vi "FPGA-HS-Parallel-Port-Receiver.vi"() -> ()   [LabVIEW 2016]
uses:
  <vilib>/Platform/TimedLoop/XDataNode/timing_clust.ctl
  <vilib>/Platform/TimedLoop/XDataNode/nitl_modes.ctl
  <vilib>/Platform/TimedLoop/XDataNode/wakeup.ctl
  <vilib>/rvi/Emulation/niFpgaGetClockAttributes.vi
  <vilib>/rvi/Emulation/niFpgaSctlEmulationGetInTimedLoop.vi
  <vilib>/rvi/Emulation/niFpgaEmulationReportErrorSimple.vi
  <vilib>/rvi/Emulation/niFpgaCriticalErrorInLSC.vi
  <vilib>/rvi/eio/common/nirviEmuTemplateMethod_errors.vi
  <vilib>/rvi/interface/RandomDataEmulation/niFpgaRandomDataHandleErrors.vi
  <vilib>/Platform/TimedLoop/XDataNode/XDataNode.xnode
  <vilib>/eio/EIONode/EIONode.xnode
  <vilib>/rvi/DataTransferAndStorage/Container/XNode/niFpgaContainer.xnode
  <vilib>/rvi/interface/RandomDataEmulation/nirviRandomDataFpgaReadWriteTemplate.vi
  <vilib>/Platform/TimedLoop/XDataNode/XDNodeRunTimeDep.lvlib
panel:
  out "CompareVal":u16
  out "OldVal":u16
  in  "StepSize":u16=1
  in  "CompArray":u16[](array[numeric])=[0, 1, 2, 3, 4, 5, 6, 7, 8, 9, 10, 11, 12, 13, 14, 15, 16, 17, 18, 19, 20, 21, 22, 23, 24, 25, 26, 27, 28, 29, 30, 31, 32, 33, 34, 35, 36, 37, 38, 39, 40, 41, 42, 43, 44, 45, 46, 47, 48, 49, 50, 51, 52, 53, 54, 55, 56, 57, 58, 59, 60, 61, 62, 63] format="%x"
  in  "StopOnError?":bool
  out "CurrentIndex":u16 format="%x"
  out "CurrentSample":u16 format="%x"
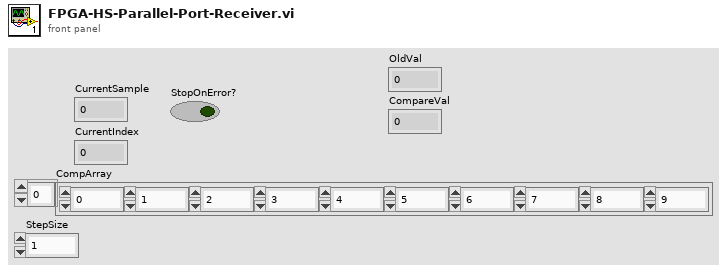
[diagram p1: front panel]
types:
  T1 = typedef "XDNodeRunTimeDep.lvlib/timing_clust.ctl" = cluster{"Expected End [f-1]":u64, "Actual End [f-1]":u64, "Finished Late? [f-1]":bool, "Expected End [i-1]":u64, "Actual End [i-1]":u64, "Finished Late? [i-1]":bool, "Expected Start [i]":u64, "Actual Start [i]":u64, "Expected Start [f]":u64, "Actual Start [f]":u64, "Source Name":string, "Structure Name":string, "Period":i64, "Deadline":i64, "Offset":i64, "Start":i64, "Priority":i32, "Timeout":i32, "Mode":T2, "Wakeup Reason":T3, "Error":errorcluster, "Source Type":string, "Secondary Source Type":string, "Global End Time":u64, "Global Start Time":u64, "Frame Duration":u64, "Iteration Duration":u64, "Assigned CPU":i32, "I/O Scan Engine Mode":u32}
  T2 = typedef "XDNodeRunTimeDep.lvlib/nitl_modes.ctl" = enum32{"No Change", "Process missed periods, maintain original phase", "Discard missed periods, maintain original phase", "Process missed periods, ignore original phase", "Discard missed periods, ignore original phase"}
  T3 = typedef "XDNodeRunTimeDep.lvlib/wakeup.ctl" = enum32{"Normal", "Aborted", "Asynchronous wakeup", "Timing source error", "Timed loop error", "Timeout"}
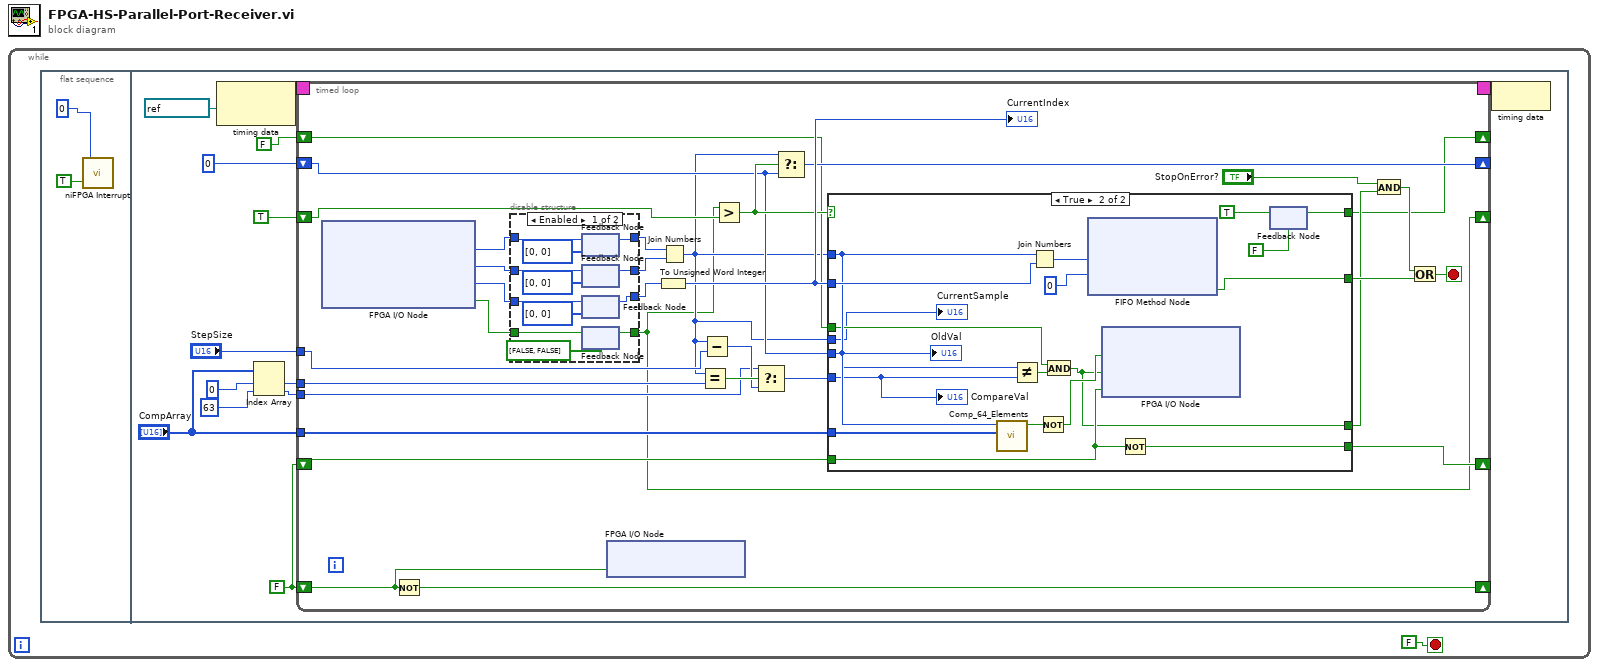
[diagram p0: block diagram]
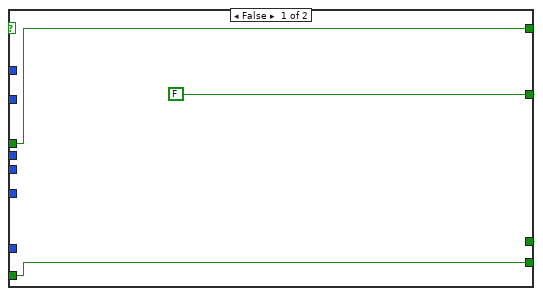
[diagram p3: hidden frame]
diagram:
  n1 = while {
    stop <- FALSE stop-if-true
    n2 = flat-sequence {
      frame #0 {
        n3 = call <vilib>:"niFPGA Interrupt.vi"("Wait Until Cleared (F)"=TRUE, "IRQ Number (0)"=u8 0) -> ()  [unwired: 1 in]
      }
      frame #1 {
        w4 = FALSE ("ConnectorB/DIO8")
        n4 = node-c288(refnum<k21> "30MHz" ("Source Name")) -> (w16:T1)
        n5 = Index Array(array="CompArray", index #1=0 ("index"), index #2=63 ("index")) -> (element #1=w8:u16, element #2=w7:u16)
        n6 = timed-loop {
          timing: w16 -> [_]
          timing-out: [_] -> w15
          shift-right: [w17] -> _
          shift-left: TRUE ("ConnectorB/DIO8") -> [w47]
          shift-right: [w46] -> _
          shift-left: w4 -> [w40]
          tunnel: "CompArray" -> [w38]
          tunnel: "StepSize" -> [w35]
          shift-right: [w32] -> _
          shift-left: u16 0 -> [w30]
          tunnel: w8 -> [w34]
          tunnel: w7 -> [w33]
          shift-right: [w28] -> _
          shift-left: FALSE -> [w29]
          shift-right: [w26] -> _
          shift-left: w4 -> [w27]
          stop <- w45 stop-if-true
          n7 = xnode "FPGA I/O Node"() -> ("ConnectorA/DIO15:8"=w24:u8, "ConnectorA/DIO7:0"=w22:u8, "ConnectorB/DIO7:0"=w19:u8, "ConnectorB/DIO8"=w18:bool)  [unwired: 4 in, 4 out]
          n8 = Not(x=w40) -> (.not. x?=w46:bool)
          n9 = disable-structure shown="Enabled" {
            disable-tunnel: w24 -> [w60 w64]
            disable-tunnel: w22 -> [w59 w63]
            disable-tunnel: w19 -> [w58 w62]
            disable-tunnel: w18 -> [w57 w61]
            disable-tunnel: [w56 w64] -> w23
            disable-tunnel: [w55 w63] -> w21
            disable-tunnel: [w54 w62] -> w20
            disable-tunnel: [w53 w61] -> w17
            frame Enabled {
              n10 = feedback #1(u8[] [0, 0]) -> (w56:u8)
              n11 = feedback-in #1(w60) -> ()
              n12 = feedback #2(u8[] [0, 0]) -> (w55:u8)
              n13 = feedback-in #2(w59) -> ()
              n14 = feedback #3(u8[] [0, 0]) -> (w54:u8)
              n15 = feedback-in #3(w58) -> ()
              n16 = feedback #4(bool[] [FALSE, FALSE]) -> (w53:bool)
              n17 = feedback-in #4(w57) -> ()
            }
            frame Disabled {
            }
          }
          n18 = xnode "FPGA I/O Node"("ConnectorC/DIO7"=w40) -> ()  [unwired: 1 in, 1 out]
          n19 = To Unsigned Word Integer(number=w20) -> (unsigned 16bit integer=w42:u16)
          "CurrentIndex" <- w42
          n20 = Join Numbers(hi=w23, lo=w21) -> ((hi.lo)=w25:u16)
          n21 = Equal?(x=w25, y=w34) -> (x = y?=w37:bool)
          n22 = Subtract(x=w25, y=w35) -> (x-y=w36:u16)
          n23 = Greater?(x=w17, y=w47) -> (0:w31:bool)
          n24 = Select(t=w33, s=w37, f=w36) -> (s? t:f=w39:u16)
          n25 = Select(t=w25, s=w31, f=w30) -> (s? t:f=w32:u16)
          n26 = case shown="True" w31 {
            tunnel: [w67 w86] -> w48
            tunnel: [w67 w72] -> w41
            tunnel: w25 -> [_ w79]
            tunnel: w42 -> [_ w83]
            tunnel: w38 -> [_ w81]
            tunnel: w39 -> [_ w77]
            tunnel: w30 -> [_ w78]
            tunnel: w29 -> [w66 w75]
            tunnel: [w66 w70] -> w28
            tunnel: w27 -> [w65 w73]
            tunnel: [w65 w74] -> w26
            tunnel: w25 -> [_ w68]
            frame False {
              w67 = FALSE ("Timed Out?")
            }
            frame True {
              n27 = call "Comp_64_Elements.vi"("Array"=w81, "CompVal"=w79) -> ("Boolean"=w85:bool)  [unwired: 9 in]
              n28 = Not Equal?(x=w78, y=w77) -> (x != y?=w76:bool)
              n29 = Join Numbers(hi=w79, lo=w83) -> ((hi.lo)=w82:u32)
              n30 = Not(x=w85) -> (.not. x?=w84:bool)
              n31 = And(x=w75, y=w76) -> (x .and. y?=w72:bool)
              n32 = xnode ("FIFO Method Node")("Element"=w82, "Timeout"=0) -> ("Timed Out?"=w86:bool)  [unwired: 1 in, 1 out]
              n33 = xnode "FPGA I/O Node"("ConnectorC/DIO0"=w84, "ConnectorC/DIO1"=w72, "ConnectorC/DIO2"=w73) -> ()  [unwired: 3 in, 3 out]
              n34 = Not(x=w73) -> (.not. x?=w74:bool)
              n35 = feedback-in #5(TRUE) -> ()
              n36 = feedback #5(FALSE) -> (w70:bool)
              "CurrentSample" <- w68
              "OldVal" <- w78
              "CompareVal" <- w77
            }
          }
          n37 = And(x="StopOnError?", y=w41) -> (x .and. y?=w44:bool)
          n38 = Or(x=w44, y=w48) -> (x .or. y?=w45:bool)
        }
        n39 = node-c288(w15) -> ()
      }
    }
  }
